vi "Intan_Create_and_OpenBinaryDatafile.vi"() -> (2 "file path":path, 3 "refnum out":refnum<file>, 4 "error out":errorcluster)   [LabVIEW 2015]
doc: "Use this VI to select path for binary data, create and open it (or replace with confirmation)"
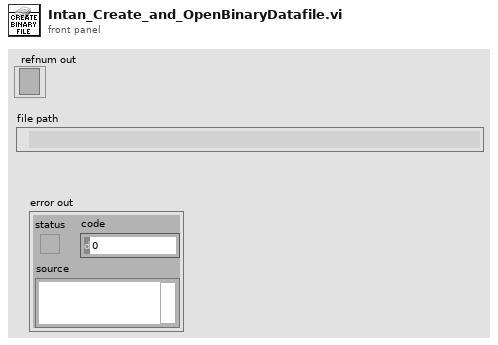
[diagram p1: front panel]
types:
  T1 = enum16{"open", "replace", "create", "open or create", "replace or create", "replace or create with confirmation"}
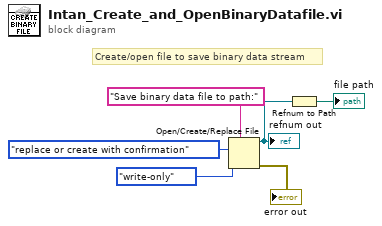
[diagram p0: block diagram]
diagram:
  # "Create/open file to save binary data stream"
  n1 = Open/Create/Replace File(prompt="Save binary data file to path:" ("prompt (Choose or enter file path)"), operation (0:open)=T1."replace or create with confirmation", access (0:read/write)=enum16{"read/write", "read-only", "write-only"}."write-only") -> (refnum out=w2:refnum<file>, error out=→"error out":errorcluster)  [unwired: 3 in, 1 out]
  "refnum out" <- w2
  n2 = Refnum to Path(1:w2) -> (0:→"file path":path)
